vi "CRYGet Upper Step Data.vi"(10 "Type In":enum16{"Curves", "Values", "Results", "WFM"}(ring), 11 "No.VI":i32) -> (0 "Waveform Array":T3 {"Y dB ref" format="%.1f"; "Y axis" items=["Log", "Lin"]; "Y data" items=["dB", "Lin"]; "X data" items=["dB", "Lin"]}, 1 "Result array":T5 {"Margin" format="%.2f"}, 2 "Value array":T1 {"Z data" items=["dB", "Lin"]; "X data" items=["dB", "Lin"]; "Y data" items=["dB", "Lin"]; "Z dB ref" format="%.1f"; "Z axis" items=["Log", "Lin"]; "X dB ref" format="%.1f"; "X axis" items=["Log", "Lin"]; "Y axis" items=["Log", "Lin"]; "Y dB ref" format="%.1f"; "Curve"."z" format="%.2f"; "Curve"."y" format="%.2f"; "Curve"."x" format="%.2f"}, 3 "Curve array":T1 {"Z data" items=["dB", "Lin"]; "X data" items=["dB", "Lin"]; "Y data" items=["dB", "Lin"]; "Z dB ref" format="%.1f"; "Z axis" items=["Log", "Lin"]; "X dB ref" format="%.1f"; "X axis" items=["Log", "Lin"]; "Y axis" items=["Log", "Lin"]; "Y dB ref" format="%.1f"; "Curve"."z" format="%.2f"; "Curve"."y" format="%.2f"; "Curve"."x" format="%.2f"})   [LabVIEW 2013]
uses:
  CRYSystem/Typedef Control/CRYData Cluster Array.ctl
  CRYSystem/Typedef Control/CRYData Cluster.ctl
  CRYSystem/Typedef Control/CRYResult Cluster Array.ctl
  CRYSystem/Typedef Control/CRYResult Cluster.ctl
  CRYSystem/Typedef Control/CRYWaveform Cluster Array.ctl
  CRYSystem/Typedef Control/CRYWaveform Cluster.ctl
  CRYProject/CRYProject Editor Global.vi
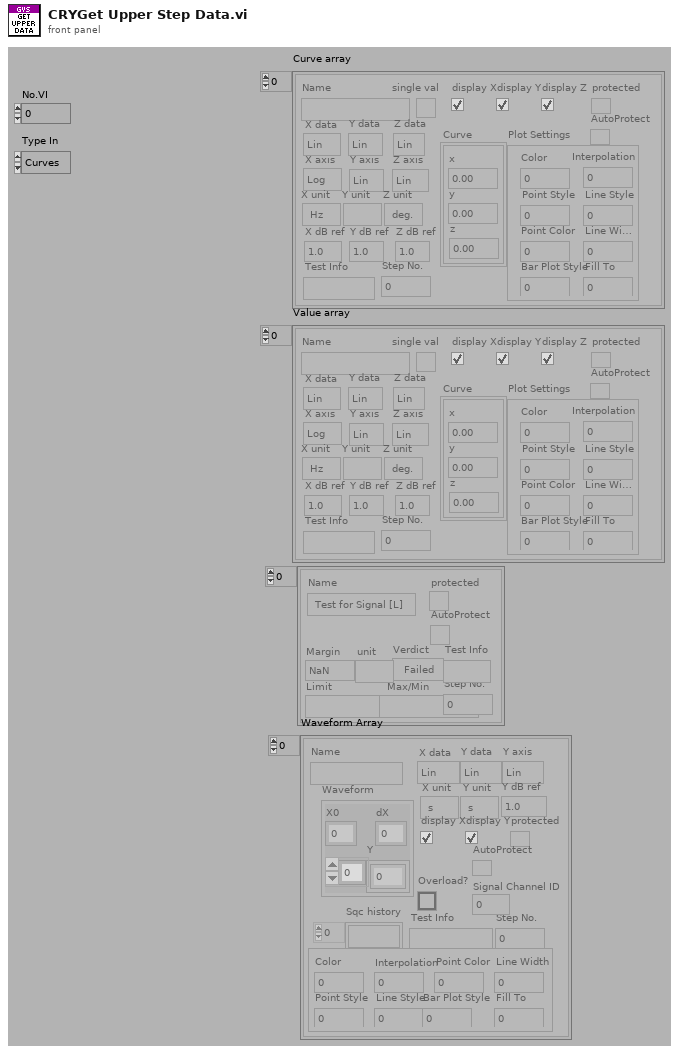
[diagram p1: front panel]
types:
  T1 = typedef "CRYData Cluster Array.ctl" = T2[]
  T2 = typedef "CRYData Cluster.ctl" = cluster{"Name":string, "Curve":cluster{"x":dbl, "y":dbl, "z":dbl}[], "X data":u16, "Y data":u16, "Z data":u16, "X axis":u16, "Y axis":u16, "Z axis":u16, "X unit":string, "Y unit":string, "Z unit":string, "X dB ref":dbl, "Y dB ref":dbl, "Z dB ref":dbl, "single val":bool, "protected":bool, "display X":bool, "display Y":bool, "display Z":bool, "Test Info":string, "Step No.":i32, "Plot Settings":cluster{"Color":u32, "Interpolation":u8, "Point Style":u8, "Line Style":u8, "Point Color":u32, "Line Width":u8, "Bar Plot Style":u8, "Fill To":i16}, "AutoProtect":bool}
  T3 = typedef "CRYWaveform Cluster Array.ctl" = T4[]
  T4 = typedef "CRYWaveform Cluster.ctl" = cluster{"Waveform":cluster{"X0":dbl, "dX":dbl, "Y":sgl[]}, "X data":u16, "Y data":u16, "Y axis":u16, "X unit":string, "Y unit":string, "Y dB ref":dbl, "display Y":bool, "display X":bool, "Overload?":bool, "Test Info":string, "Step No.":i32, "Name":string, "protected":bool, "Sqc history":string[], "Signal Channel ID":i32, "Plot Settings":cluster{"Color":u32, "Interpolation":u8, "Point Style":u8, "Line Style":u8, "Point Color":u32, "Line Width":u8, "Bar Plot Style":u8, "Fill To":i16}, "AutoProtect":bool}
  T5 = typedef "CRYResult Cluster Array.ctl" = T6[]
  T6 = typedef "CRYResult Cluster.ctl" = cluster{"Name":string, "Margin":dbl, "unit":string, "Verdict":bool, "Limit":string, "Max/Min":string, "protected":bool, "Step No.":i32, "Test Info":string, "AutoProtect":bool}
  T7 = typedef "CRYStep.ctl" = cluster{"No.VI":i32, "Category":string, "StepName":string, "Seq setup flattened":string, "Comment":string, "Steps config.":bool[], "Jump config":i32[], "Start":dbl, "Increment":dbl, "Name":string, "Unit":string, "Y data":u16, "Y prefix":string, "Y dB ref":dbl, "Y unit":string, "Repeat State Array":cluster{"Start":dbl, "Increment":dbl, "Count":i32, "Num":i32}[]}
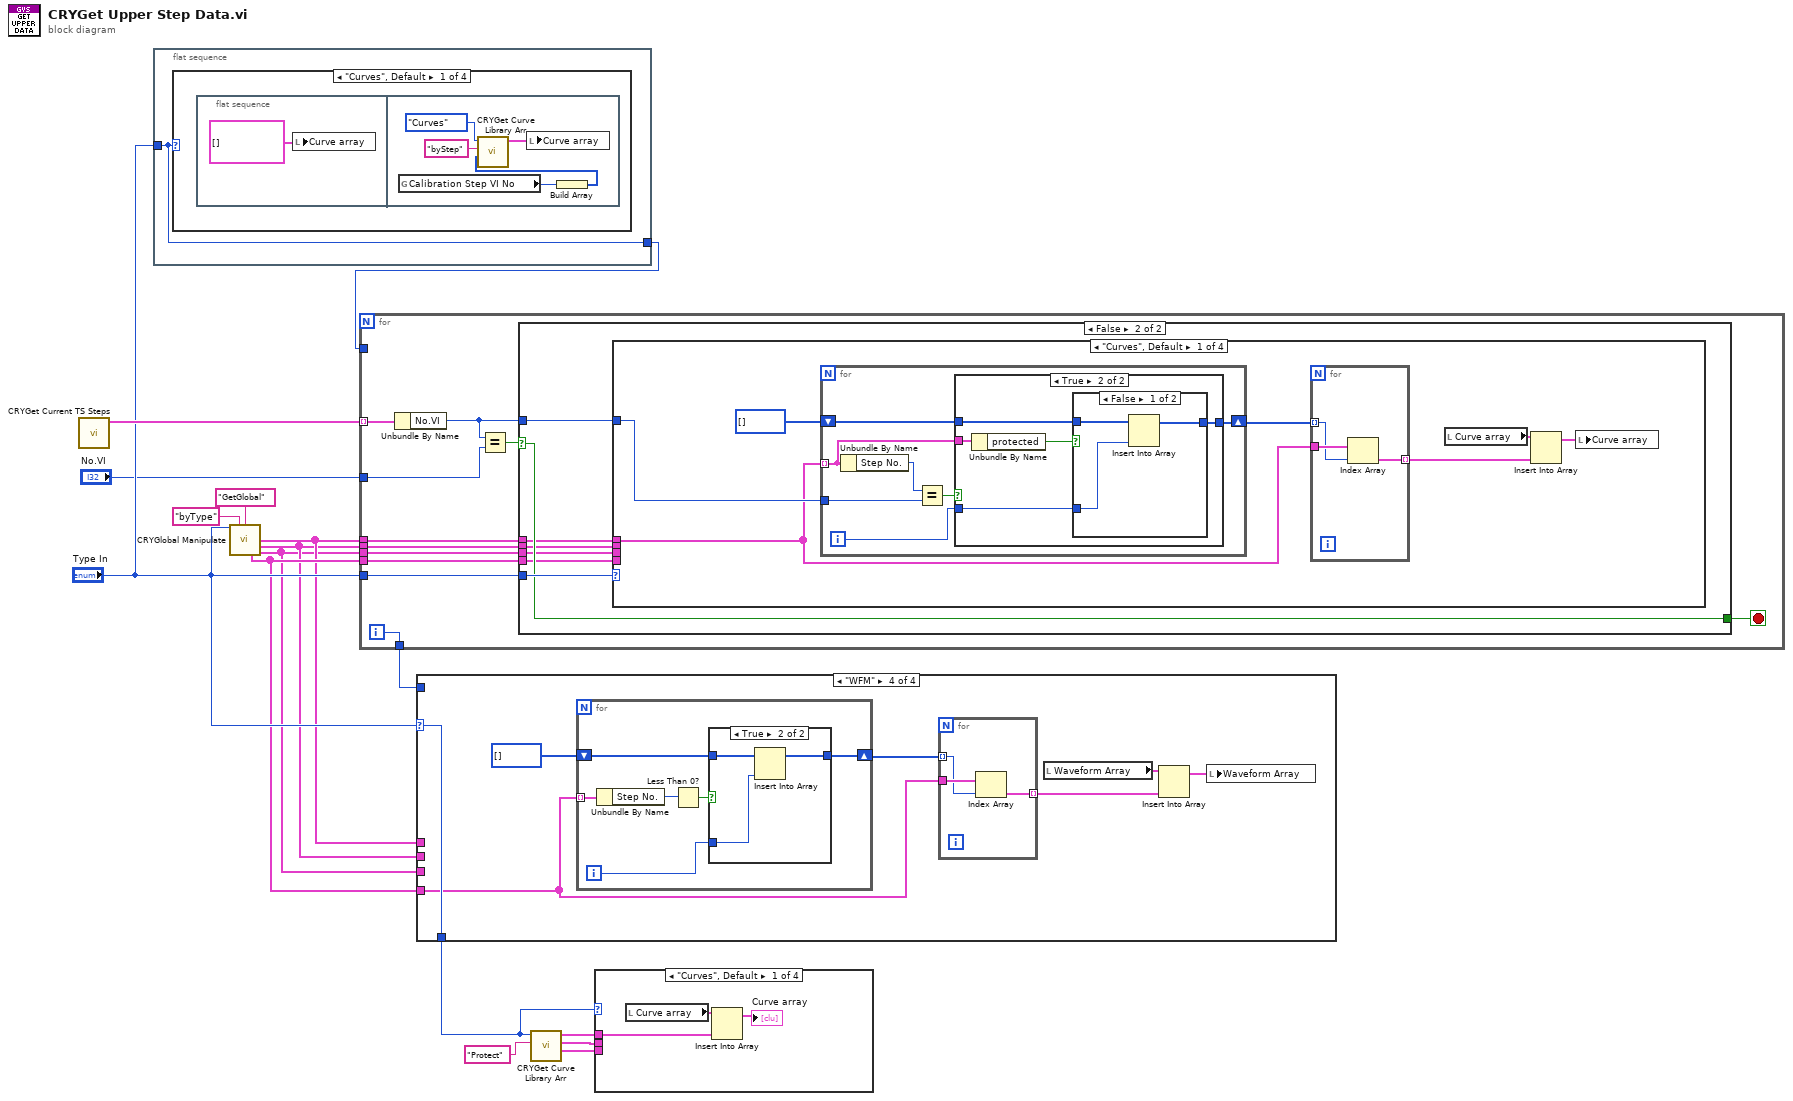
[diagram p0: block diagram]
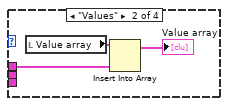
[diagram p2: hidden frame]
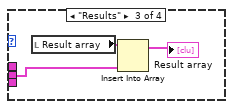
[diagram p3: hidden frame]
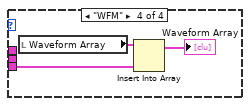
[diagram p4: hidden frame]
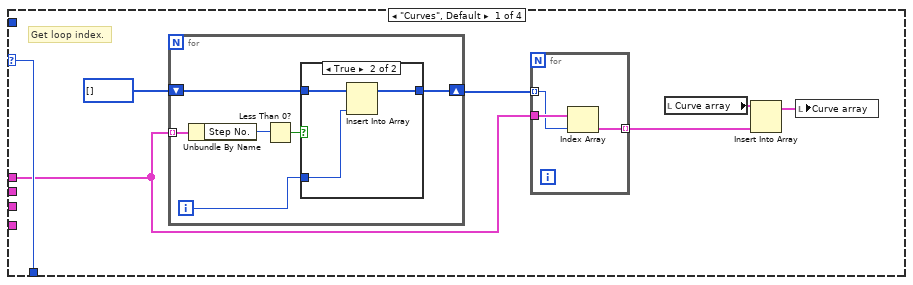
[diagram p5: hidden frame]
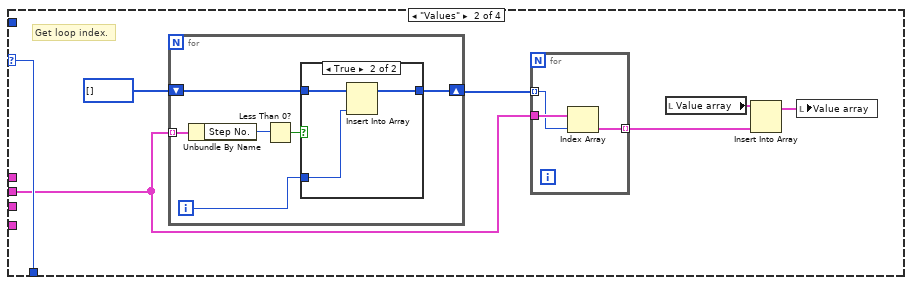
[diagram p7: hidden frame]
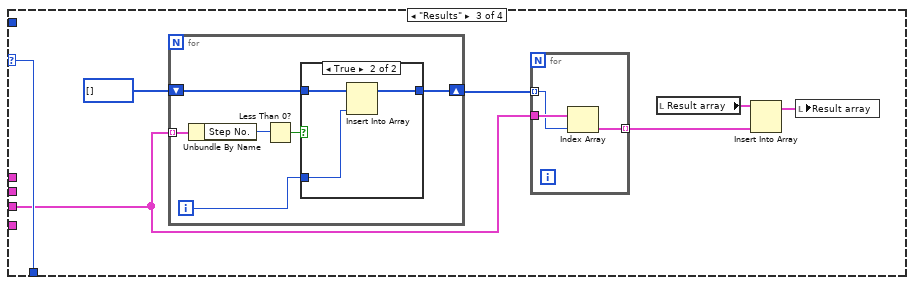
[diagram p9: hidden frame]
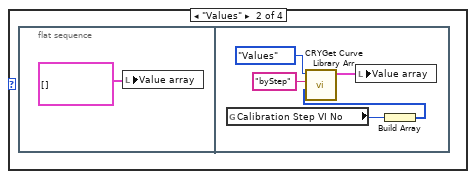
[diagram p12: hidden frame]
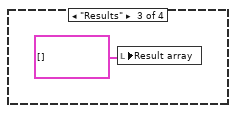
[diagram p13: hidden frame]
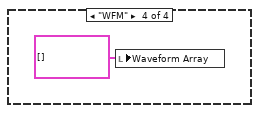
[diagram p14: hidden frame]
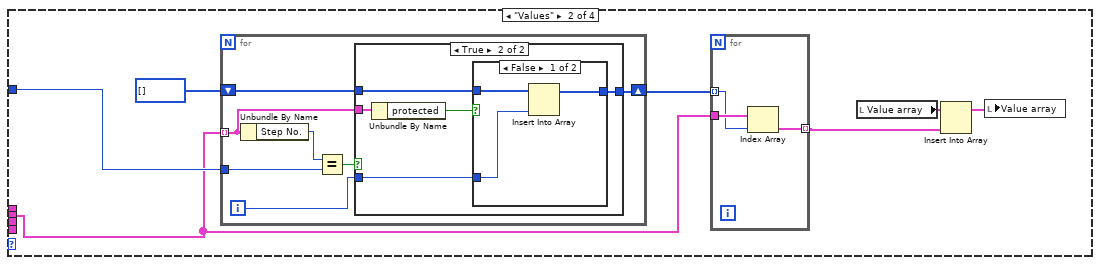
[diagram p18: hidden frame]
diagram:
  n1 = call "CRYGet Current TS Steps.vi"() -> ("Steps"=w15:T7[])  [unwired: 1 in, 10 out]
  n2 = flat-sequence {
    tunnel: "Type In" -> [w17]
    tunnel: [w17] -> w16
    frame #0 {
      n3 = case shown="\"Curves\", Default" w17 {
        frame "Curves", Default {
          n4 = flat-sequence {
            frame #0 {
              n5 = local write "Curve array"(T1 [] ("Curve array")) -> ()
            }
            frame #1 {
              n6 = global read "CRYProject Editor Global.vi" "Calibration Step VI No"() -> (w21:i32)
              n7 = Build Array(w21) -> (w20:i32[])
              n8 = call "CRYGet Curve Library Arr.vi"("Index"=w20, "sOption"="byStep", "Type In"=enum16{"Curves", "Values", "Results", "WFM"}."Curves") -> ("Curves/Values"=w23:T1)  [unwired: 6 in, 2 out]
              n9 = local write "Curve array"(w23) -> ()
            }
          }
        }
        frame "Values" {
          n10 = flat-sequence {
            frame #0 {
              n11 = local write "Value array"(T1 [] ("Curve array")) -> ()
            }
            frame #1 {
              n12 = global read "CRYProject Editor Global.vi" "Calibration Step VI No"() -> (w27:i32)
              n13 = Build Array(w27) -> (w26:i32[])
              n14 = call "CRYGet Curve Library Arr.vi"("Index"=w26, "sOption"="byStep", "Type In"=enum16{"Curves", "Values", "Results", "WFM"}."Values") -> ("Curves/Values"=w29:T1)  [unwired: 6 in, 2 out]
              n15 = local write "Value array"(w29) -> ()
            }
          }
        }
        frame "Results" {
          n16 = local write "Result array"(T5 [] ("Result array")) -> ()
        }
        frame "WFM" {
          n17 = local write "Waveform Array"(T3 [] ("Waveform Array")) -> ()
        }
      }
    }
  }
  n18 = call "CRYGlobal Manipulate.vi"("Type"="Type In", "sOption"="byType", "sAction"="GetGlobal") -> ("Curves Out"=w4:T2[], "Values Out"=w3:T2[], "WFM Out"=w5:T4[], "Results Out"=w2:T6[])  [unwired: 6 in, 3 out]
  n19 = for {
    tunnel: w15 -> [w40] mode=indexing
    tunnel: "Type In" -> [w41]
    tunnel: w16 -> [_]
    tunnel: [w38] -> w14
    tunnel: w4 -> [w37]
    tunnel: w3 -> [w36]
    tunnel: w2 -> [w35]
    tunnel: w5 -> [w34]
    tunnel: "No.VI" -> [w33]
    i -> [w38]
    stop <- w39 stop-if-true
    n20 = Unbundle By Name(w40) -> ("No.VI"=w32:i32)
    n21 = Equal?(x=w32, y=w33) -> (x = y?=w42:bool)
    n22 = case shown="False" w42 {
      selector: w42 -> [w43 w49]
      tunnel: w41 -> [_ w50]
      tunnel: [w43 w49] -> w39
      tunnel: w32 -> [_ w48]
      tunnel: w37 -> [_ w47]
      tunnel: w36 -> [_ w46]
      tunnel: w35 -> [_ w45]
      tunnel: w34 -> [_ w44]
      frame True {
      }
      frame False {
        n23 = case shown="\"Curves\", Default" w50 {
          tunnel: w48 -> [w52 w79 w106 w133]
          tunnel: w47 -> [w51 _ _ _]
          tunnel: w46 -> [_ w78 _ _]
          tunnel: w45 -> [_ _ w105 _]
          tunnel: w44 -> [_ _ _ w132]
          frame "Curves", Default {
            n24 = for {
              tunnel: w51 -> [w62] mode=indexing
              tunnel: w52 -> [w67]
              shift-right: [w63] -> w56
              shift-left: i32[] [] -> [w65]
              i -> [w64]
              n25 = Unbundle By Name(w62) -> ("Step No."=w61:i32)
              n26 = Equal?(x=w61, y=w67) -> (x = y?=w66:bool)
              n27 = case shown="True" w66 {
                tunnel: w65 -> [w68 w73]
                tunnel: w64 -> [_ w72]
                tunnel: [w68 w71] -> w63
                tunnel: w62 -> [_ w70]
                frame False {
                }
                frame True {
                  n28 = Unbundle By Name(w70) -> ("protected"=w69:bool)
                  n29 = case shown="False" w69 {
                    tunnel: w73 -> [w76 w77]
                    tunnel: w72 -> [w75 _]
                    tunnel: [w74 w77] -> w71
                    frame False {
                      n30 = Insert Into Array(array=w76, new element=w75) -> (w74:i32[])  [unwired: 1 in]
                    }
                    frame True {
                    }
                  }
                }
              }
            }
            n31 = for {
              tunnel: w56 -> [w59] mode=indexing
              tunnel: w51 -> [w60]
              tunnel: [w58] -> w53 mode=indexing
              n32 = Index Array(array=w60, index=w59) -> (element=w58:T2)
            }
            n33 = local read "Curve array"() -> (w54:T1)
            n34 = Insert Into Array(array=w54, new element=w53) -> (w55:T1)  [unwired: 1 in]
            n35 = local write "Curve array"(w55) -> ()
          }
          frame "Values" {
            n36 = for {
              tunnel: w78 -> [w88] mode=indexing
              tunnel: w79 -> [w94]
              shift-right: [w90] -> w83
              shift-left: i32[] [] -> [w92]
              i -> [w91]
              n37 = Unbundle By Name(w88) -> ("Step No."=w89:i32)
              n38 = Equal?(x=w89, y=w94) -> (x = y?=w93:bool)
              n39 = case shown="True" w93 {
                tunnel: w92 -> [w95 w100]
                tunnel: w91 -> [_ w99]
                tunnel: [w95 w98] -> w90
                tunnel: w88 -> [_ w97]
                frame False {
                }
                frame True {
                  n40 = Unbundle By Name(w97) -> ("protected"=w96:bool)
                  n41 = case shown="False" w96 {
                    tunnel: w100 -> [w103 w104]
                    tunnel: w99 -> [w102 _]
                    tunnel: [w101 w104] -> w98
                    frame False {
                      n42 = Insert Into Array(array=w103, new element=w102) -> (w101:i32[])  [unwired: 1 in]
                    }
                    frame True {
                    }
                  }
                }
              }
            }
            n43 = for {
              tunnel: w83 -> [w86] mode=indexing
              tunnel: w78 -> [w87]
              tunnel: [w85] -> w80 mode=indexing
              n44 = Index Array(array=w87, index=w86) -> (element=w85:T2)
            }
            n45 = local read "Value array"() -> (w81:T1)
            n46 = Insert Into Array(array=w81, new element=w80) -> (w82:T1)  [unwired: 1 in]
            n47 = local write "Value array"(w82) -> ()
          }
          frame "Results" {
            n48 = for {
              tunnel: w105 -> [w115] mode=indexing
              tunnel: w106 -> [w121]
              shift-right: [w117] -> w110
              shift-left: i32[] [] -> [w119]
              i -> [w118]
              n49 = Unbundle By Name(w115) -> ("Step No."=w116:i32)
              n50 = Equal?(x=w116, y=w121) -> (x = y?=w120:bool)
              n51 = case shown="True" w120 {
                tunnel: w119 -> [w122 w127]
                tunnel: w118 -> [_ w126]
                tunnel: [w122 w125] -> w117
                tunnel: w115 -> [_ w124]
                frame False {
                }
                frame True {
                  n52 = Unbundle By Name(w124) -> ("protected"=w123:bool)
                  n53 = case shown="False" w123 {
                    tunnel: w127 -> [w130 w131]
                    tunnel: w126 -> [w129 _]
                    tunnel: [w128 w131] -> w125
                    frame False {
                      n54 = Insert Into Array(array=w130, new element=w129) -> (w128:i32[])  [unwired: 1 in]
                    }
                    frame True {
                    }
                  }
                }
              }
            }
            n55 = for {
              tunnel: w110 -> [w113] mode=indexing
              tunnel: w105 -> [w114]
              tunnel: [w112] -> w107 mode=indexing
              n56 = Index Array(array=w114, index=w113) -> (element=w112:T6)
            }
            n57 = local read "Result array"() -> (w108:T5)
            n58 = Insert Into Array(array=w108, new element=w107) -> (w109:T5)  [unwired: 1 in]
            n59 = local write "Result array"(w109) -> ()
          }
          frame "WFM" {
            n60 = for {
              tunnel: w132 -> [w142] mode=indexing
              tunnel: w133 -> [w148]
              shift-right: [w144] -> w138
              shift-left: i32[] [] -> [w146]
              i -> [w145]
              n61 = Unbundle By Name(w142) -> ("Step No."=w143:i32)
              n62 = Equal?(x=w143, y=w148) -> (x = y?=w147:bool)
              n63 = case shown="True" w147 {
                tunnel: w146 -> [w149 w154]
                tunnel: w145 -> [_ w153]
                tunnel: [w149 w152] -> w144
                tunnel: w142 -> [_ w151]
                frame False {
                }
                frame True {
                  n64 = Unbundle By Name(w151) -> ("protected"=w150:bool)
                  n65 = case shown="False" w150 {
                    tunnel: w154 -> [w157 w158]
                    tunnel: w153 -> [w156 _]
                    tunnel: [w155 w158] -> w152
                    frame False {
                      n66 = Insert Into Array(array=w157, new element=w156) -> (w155:i32[])  [unwired: 1 in]
                    }
                    frame True {
                    }
                  }
                }
              }
            }
            n67 = for {
              tunnel: w138 -> [w140] mode=indexing
              tunnel: w132 -> [w141]
              tunnel: [w139] -> w134 mode=indexing
              n68 = Index Array(array=w141, index=w140) -> (element=w139:T4)
            }
            n69 = local read "Waveform Array"() -> (w135:T3)
            n70 = Insert Into Array(array=w135, new element=w134) -> (w136:T3)  [unwired: 1 in]
            n71 = local write "Waveform Array"(w136) -> ()
          }
        }
      }
    }
  }
  n72 = case shown="\"WFM\"" "Type In" {
    selector: "Type In" -> [w160 w180 w200 w220]
    tunnel: w14 -> [_ _ _ _]
    tunnel: [w160 w180 w200 w220] -> w13
    tunnel: w5 -> [_ _ _ w219]
    tunnel: w4 -> [w159 _ _ _]
    tunnel: w3 -> [_ w179 _ _]
    tunnel: w2 -> [_ _ w199 _]
    frame "Curves", Default {
      # "Get loop index."
      n73 = for {
        tunnel: w159 -> [w171] mode=indexing
        shift-right: [w172] -> w164
        shift-left: i32[] [] -> [w174]
        i -> [w173]
        n74 = Unbundle By Name(w171) -> ("Step No."=w170:i32)
        n75 = Less Than 0?(x=w170) -> (x < 0?=w169:bool)
        n76 = case shown="True" w169 {
          tunnel: w174 -> [w175 w178]
          tunnel: [w175 w177] -> w172
          tunnel: w173 -> [_ w176]
          frame False {
          }
          frame True {
            n77 = Insert Into Array(array=w178, new element=w176) -> (w177:i32[])  [unwired: 1 in]
          }
        }
      }
      n78 = for {
        tunnel: w164 -> [w167] mode=indexing
        tunnel: w159 -> [w168]
        tunnel: [w166] -> w161 mode=indexing
        n79 = Index Array(array=w168, index=w167) -> (element=w166:T2)
      }
      n80 = local read "Curve array"() -> (w162:T1)
      n81 = Insert Into Array(array=w162, new element=w161) -> (w163:T1)  [unwired: 1 in]
      n82 = local write "Curve array"(w163) -> ()
    }
    frame "Values" {
      # "Get loop index."
      n83 = for {
        tunnel: w179 -> [w191] mode=indexing
        shift-right: [w192] -> w184
        shift-left: i32[] [] -> [w194]
        i -> [w193]
        n84 = Unbundle By Name(w191) -> ("Step No."=w190:i32)
        n85 = Less Than 0?(x=w190) -> (x < 0?=w189:bool)
        n86 = case shown="True" w189 {
          tunnel: w194 -> [w195 w198]
          tunnel: [w195 w197] -> w192
          tunnel: w193 -> [_ w196]
          frame False {
          }
          frame True {
            n87 = Insert Into Array(array=w198, new element=w196) -> (w197:i32[])  [unwired: 1 in]
          }
        }
      }
      n88 = for {
        tunnel: w184 -> [w187] mode=indexing
        tunnel: w179 -> [w188]
        tunnel: [w186] -> w181 mode=indexing
        n89 = Index Array(array=w188, index=w187) -> (element=w186:T2)
      }
      n90 = local read "Value array"() -> (w182:T1)
      n91 = Insert Into Array(array=w182, new element=w181) -> (w183:T1)  [unwired: 1 in]
      n92 = local write "Value array"(w183) -> ()
    }
    frame "Results" {
      n93 = for {
        tunnel: w199 -> [w211] mode=indexing
        shift-right: [w212] -> w204
        shift-left: i32[] [] -> [w214]
        i -> [w213]
        n94 = Unbundle By Name(w211) -> ("Step No."=w210:i32)
        n95 = Less Than 0?(x=w210) -> (x < 0?=w209:bool)
        n96 = case shown="True" w209 {
          tunnel: w214 -> [w215 w218]
          tunnel: [w215 w217] -> w212
          tunnel: w213 -> [_ w216]
          frame False {
          }
          frame True {
            n97 = Insert Into Array(array=w218, new element=w216) -> (w217:i32[])  [unwired: 1 in]
          }
        }
      }
      n98 = for {
        tunnel: w204 -> [w207] mode=indexing
        tunnel: w199 -> [w208]
        tunnel: [w206] -> w201 mode=indexing
        n99 = Index Array(array=w208, index=w207) -> (element=w206:T6)
      }
      n100 = local read "Result array"() -> (w202:T5)
      n101 = Insert Into Array(array=w202, new element=w201) -> (w203:T5)  [unwired: 1 in]
      n102 = local write "Result array"(w203) -> ()
    }
    frame "WFM" {
      n103 = for {
        tunnel: w219 -> [w231] mode=indexing
        shift-right: [w232] -> w224
        shift-left: i32[] [] -> [w234]
        i -> [w233]
        n104 = Unbundle By Name(w231) -> ("Step No."=w230:i32)
        n105 = Less Than 0?(x=w230) -> (x < 0?=w229:bool)
        n106 = case shown="True" w229 {
          tunnel: w234 -> [w235 w238]
          tunnel: [w235 w237] -> w232
          tunnel: w233 -> [_ w236]
          frame False {
          }
          frame True {
            n107 = Insert Into Array(array=w238, new element=w236) -> (w237:i32[])  [unwired: 1 in]
          }
        }
      }
      n108 = for {
        tunnel: w224 -> [w227] mode=indexing
        tunnel: w219 -> [w228]
        tunnel: [w226] -> w221 mode=indexing
        n109 = Index Array(array=w228, index=w227) -> (element=w226:T4)
      }
      n110 = local read "Waveform Array"() -> (w222:T3)
      n111 = Insert Into Array(array=w222, new element=w221) -> (w223:T3)  [unwired: 1 in]
      n112 = local write "Waveform Array"(w223) -> ()
    }
  }
  n113 = call "CRYGet Curve Library Arr.vi"("sOption"="Protect", "Type In"=w13) -> ("Waveforms"=w9:T3, "Results"=w10:T5, "Curves/Values"=w12:T1)  [unwired: 1 in, 6 out]
  n114 = case shown="\"Curves\", Default" w13 {
    tunnel: w12 -> [w240 w243 _ _]
    tunnel: w10 -> [_ _ w246 _]
    tunnel: w9 -> [_ _ _ w249]
    frame "Curves", Default {
      n115 = local read "Curve array"() -> (w241:T1)
      n116 = Insert Into Array(array=w241, new element=w240) -> (→"Curve array":T1)  [unwired: 1 in]
    }
    frame "Values" {
      n117 = local read "Value array"() -> (w244:T1)
      n118 = Insert Into Array(array=w244, new element=w243) -> (→"Value array":T1)  [unwired: 1 in]
    }
    frame "Results" {
      n119 = local read "Result array"() -> (w247:T5)
      n120 = Insert Into Array(array=w247, new element=w246) -> (→"Result array":T5)  [unwired: 1 in]
    }
    frame "WFM" {
      n121 = local read "Waveform Array"() -> (w250:T3)
      n122 = Insert Into Array(array=w250, new element=w249) -> (→"Waveform Array":T3)  [unwired: 1 in]
    }
  }
